vi "RT (Top Level).vi"() -> ()   [LabVIEW 2017]
doc: "This is the main application launcher VI.\n\nIt is used to create the shutdown user event and launch system modules."
uses:
  User Events/TypeDefs/Shutdown UE FGV Command.ctl
  <vilib>/event_ctls.llb/usereventprio.ctl
  Modules/WinHost/WinHost.lvlib
  Modules/Controller/Controller.lvlib
  Modules/Error Handler/Error Handler.lvlib
  modules/Game/Game.lvlib
  Modules/Logger/Logger.lvlib
  modules/mypam/myPAM.lvlib
panel:
  out "error out":errorcluster
  in  "Stop RT":bool
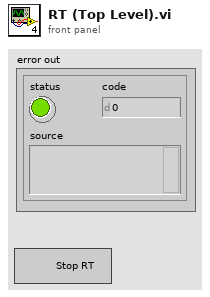
[diagram p1: front panel]
types:
  T1 = typedef "Shutdown UE FGV Command.ctl" = enum16{"create", "get", "destroy"}
  T2 = typedef "usereventprio.ctl" = enum32{"high priority", "normal priority"}
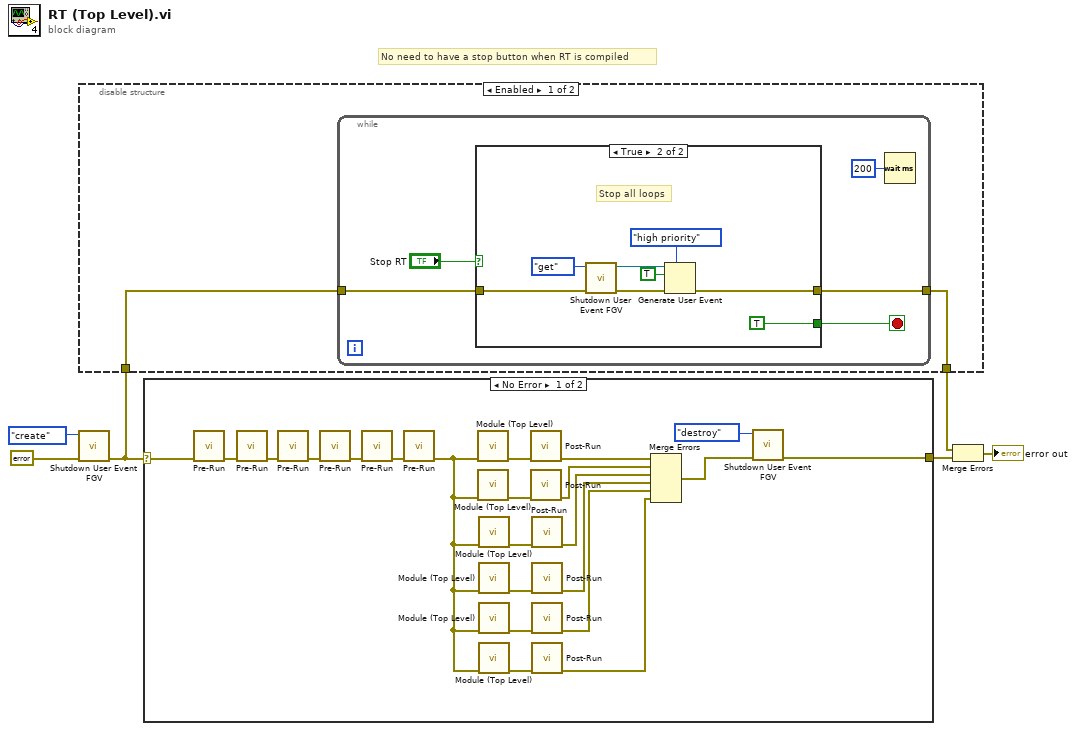
[diagram p0: block diagram]
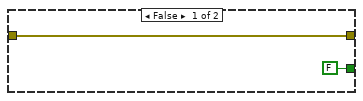
[diagram p2: hidden frame]
diagram:
  # "No need to have a stop button when RT is compiled"
  n1 = call "Shutdown User Event FGV.vi"("error in"=errorcluster {"status"=FALSE, "code"=0, "source"=""} ("Error In"), "command"=Shutdown_UE_FGV_Command."create" ("Command")) -> ("error out"=w4:errorcluster)  [unwired: 8 in, 1 out]
  n2 = disable-structure shown="Enabled" {
    disable-tunnel: w4 -> [w8 w24]
    disable-tunnel: [w7 w24] -> w3
    frame Enabled {
      n3 = while {
        tunnel: w8 -> [w11]
        tunnel: [w9] -> w7
        stop <- w10 stop-if-true
        n4 = case shown="True" "Stop RT" {
          tunnel: w11 -> [w14 w18]
          tunnel: [FALSE TRUE] -> w10
          tunnel: [w14 w16] -> w9
          frame False {
          }
          frame True {
            # "Stop all loops"
            n5 = call "Shutdown User Event FGV.vi"("error in"=w18, "command"=Shutdown_UE_FGV_Command."get" ("Command")) -> ("error out"=w21:errorcluster, "shutdown user event"=w22:refnum<user-event>)  [unwired: 8 in]
            n6 = Generate User Event(priority (normal)=usereventprio."high priority", user event=w22, event data cluster=TRUE ("event data"), error in=w21) -> (error out=w16:errorcluster)  [unwired: 1 out]
          }
        }
        n7 = Wait (ms)(milliseconds to wait=u32 200) -> ()  [unwired: 1 out]
      }
    }
    frame Disabled {
    }
  }
  n8 = case shown="No Error" w4 {
    selector: w4 -> [w43 w47]
    tunnel: [w45 w47] -> w5
    frame No Error {
      n9 = call "Pre-Run.vi"("error in"=w43) -> ("error out"=w42:errorcluster)  [unwired: 10 in]
      n10 = call "Pre-Run.vi"("error in"=w42) -> ("error out"=w41:errorcluster)  [unwired: 10 in]
      n11 = call "Pre-Run.vi"("error in"=w41) -> ("error out"=w40:errorcluster)  [unwired: 10 in]
      n12 = call "Pre-Run.vi"("error in"=w40) -> ("error out"=w39:errorcluster)  [unwired: 10 in]
      n13 = call "Pre-Run.vi"("error in"=w39) -> ("error out"=w38:errorcluster)  [unwired: 10 in]
      n14 = call "Pre-Run.vi"("error in"=w38) -> ("error out"=w37:errorcluster)  [unwired: 10 in]
      n15 = call "Module (Top Level).vi"("error in"=w37) -> ("error out"=w36:errorcluster)  [unwired: 10 in]
      n16 = call "Module (Top Level).vi"("error in"=w37) -> ("error out"=w35:errorcluster)  [unwired: 10 in]
      n17 = call "Module (Top Level).vi"("error in"=w37) -> ("error out"=w25:errorcluster)  [unwired: 10 in]
      n18 = call "Module (Top Level).vi"("error in"=w37) -> ("error out"=w34:errorcluster)  [unwired: 10 in]
      n19 = call "Module (Top Level).vi"("error in"=w37) -> ("error out"=w33:errorcluster)  [unwired: 10 in]
      n20 = call "Module (Top Level).vi"("error in"=w37) -> ("error out"=w32:errorcluster)  [unwired: 10 in]
      n21 = call "Post-Run.vi"("error in"=w36) -> ("error out"=w31:errorcluster)  [unwired: 10 in]
      n22 = call "Post-Run.vi"("error in"=w35) -> ("error out"=w30:errorcluster)  [unwired: 10 in]
      n23 = call "Post-Run.vi"("error in"=w25) -> ("error out"=w29:errorcluster)  [unwired: 10 in]
      n24 = call "Post-Run.vi"("error in"=w34) -> ("error out"=w28:errorcluster)  [unwired: 10 in]
      n25 = call "Post-Run.vi"("error in"=w33) -> ("error out"=w27:errorcluster)  [unwired: 10 in]
      n26 = call "Post-Run.vi"("error in"=w32) -> ("error out"=w26:errorcluster)  [unwired: 10 in]
      n27 = Merge Errors(w31, w30, w29, w28, w27, w26) -> (w44:errorcluster)
      n28 = call "Shutdown User Event FGV.vi"("error in"=w44, "command"=Shutdown_UE_FGV_Command."destroy" ("Command")) -> ("error out"=w45:errorcluster)  [unwired: 8 in, 1 out]
    }
    frame Error {
      # "User Event Creation Error\nDon't start the application"
    }
  }
  n29 = Merge Errors(w3, w5) -> (→"error out":errorcluster)
